vi "finalI.vi"() -> ()   [LabVIEW 2013]
panel:
  out "Array":i32[](array[numeric])
  out "appended array":i32[][](array[numeric])
  out "unsigned byte array":u8[](array[numeric])
  out "concatenated string":string
  out "we array":i32[](array[numeric])
  out "2d array sorted":i32[][](array[numeric])
  in  "stop":bool
  out "iterarions :":dbl
  out "Slide":u32(slide) scale=0.0..3000.0
  out "A letter":string
  out "B letter":string
  out "PASSWORD":string
  out "Utterance":dbl[](graph)
  out "Input Signal Energy":dbl
  out "?":bool
  out "?":bool
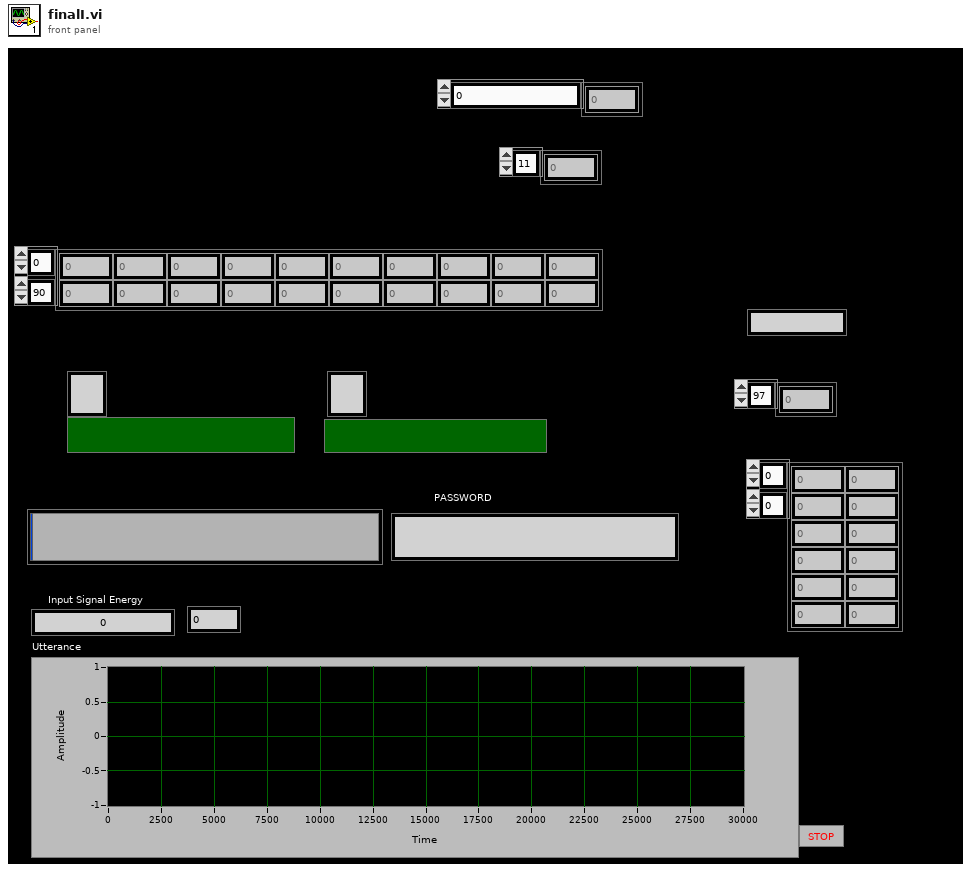
[diagram p1: front panel]
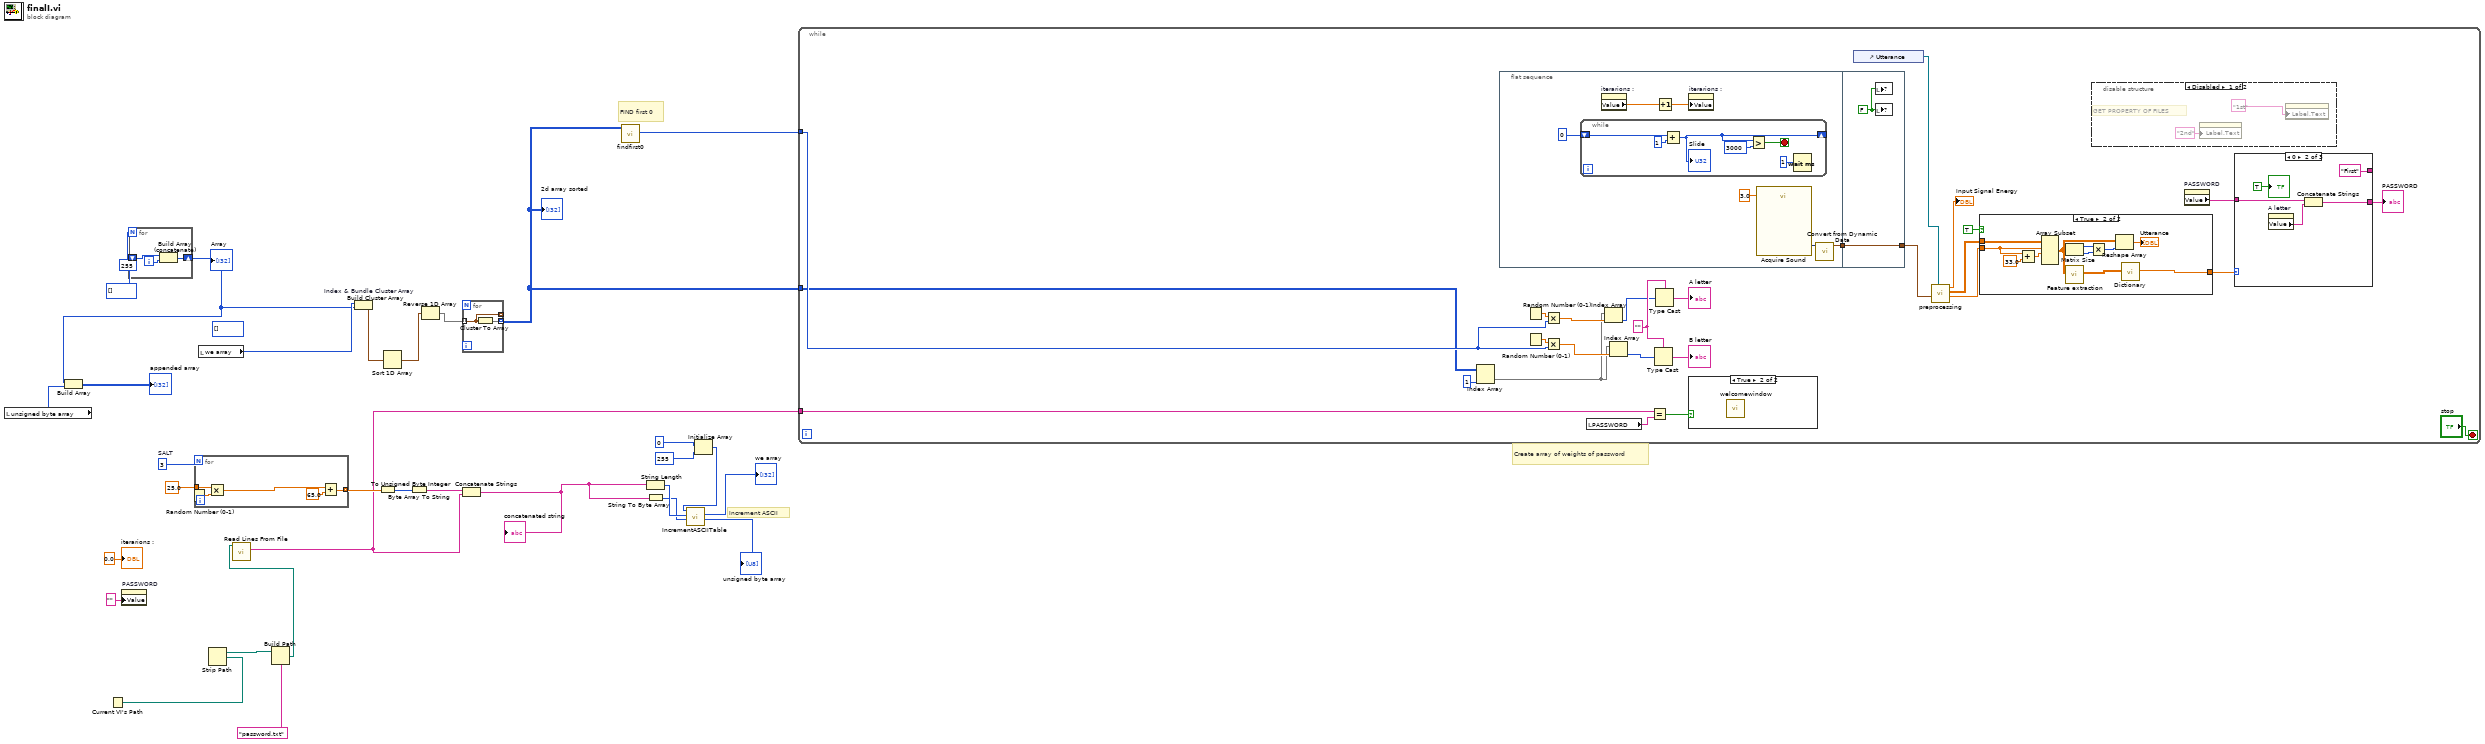
[diagram p0: block diagram]
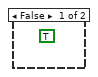
[diagram p3: hidden frame]
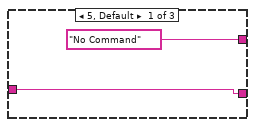
[diagram p4: hidden frame]
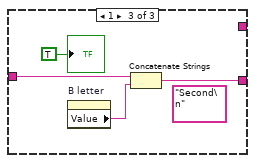
[diagram p5: hidden frame]
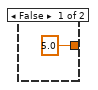
[diagram p6: hidden frame]
diagram:
  (unwired) i32[] []
  w26 = 3  # SALT
  # "FIND first 0"
  # "Create array of weights of password"
  # "Increment ASCII"
  n1 = local read "unsigned byte array"() -> (w9:u8[])
  n2 = Current VI's Path() -> (path=w4:path)
  n3 = property on="PASSWORD" class="Str"("Value"="" ("PASSWORD")) -> ()  [unwired: 2 in, 2 out]
  n4 = for {
    N: 255 -> [_]
    shift-right: [w31] -> w10
    shift-left: i32[] [] -> [w33]
    i -> [w32]
    n5 = Build Array (concatenate)(w33, w32) -> (w31:i32[])
  }
  "Array" <- w10
  n6 = Build Array(w10, w9) -> (→"appended array":i32[][])
  n7 = for {
    N: w26 -> [_]
    tunnel: 25.0 -> [w35]
    tunnel: [w34] -> w28 mode=indexing
    n8 = Random Number (0-1)() -> (number: 0 to 1=w38:dbl)
    n9 = Multiply(x=w35, y=w38) -> (x*y=w36:dbl)
    n10 = Add(x=w36, y=65.0) -> (x+y=w34:dbl)
  }
  n11 = local read "we array"() -> (w14:i32[])
  n12 = Strip Path(path=w4) -> (stripped path=w3:path)  [unwired: 1 out]
  n13 = Build Path(base path=w3, name or relative path="password.txt") -> (appended path=w1:path)
  n14 = call <vilib>:"Read Lines From File.vi"("file path (dialog if empty)"=w1) -> ("line string"=w5:string)  [unwired: 5 in, 3 out]
  n15 = Build Cluster Array "Index & Bundle Cluster Array"(w14, w10) -> (w15:cluster{"dimension size":i32, i32}[])
  n16 = To Unsigned Byte Integer(number=w28) -> (unsigned 8bit integer=w29:u8[])
  n17 = Sort 1D Array(array=w15) -> (sorted array=w13:cluster{"dimension size":i32, i32}[])
  n18 = Byte Array To String(unsigned byte array=w29) -> (string=w25:string)
  n19 = Reverse 1D Array(array=w13) -> (reversed array=w12:cluster{"dimension size":i32, i32}[])
  n20 = for {
    tunnel: [w39] -> _ mode=indexing
    tunnel: [w40] -> w7 mode=indexing
    tunnel: w12 -> [w39] mode=indexing
    n21 = Cluster To Array(cluster=w39) -> (array=w40:i32[])
  }
  "2d array sorted" <- w7
  n22 = Concatenate Strings(w25, w5) -> (w30:string)
  "concatenated string" <- w30
  n23 = call "findfirst0.vi"("Array"=w7) -> ("index of element"=w6:i32)  [unwired: 10 in]
  n24 = String Length(string=w30) -> (length=w24:i32)
  n25 = String To Byte Array(string=w30) -> (unsigned byte array=w21:u8[])
  "unsigned byte array" <- w21
  n26 = Initialize Array(0 ("dimension size"), 255 ("dimension size")) -> (w11:i32[])
  n27 = call "IncrementASCIITable.vi"("0255array"=w21, "Numeric"=w24, "Array in"=w11) -> ("we array"=→"we array":i32[])  [unwired: 7 in, 1 out]
  n28 = while {
    tunnel: w5 -> [w54]
    tunnel: w7 -> [w45]
    tunnel: w6 -> [w46]
    stop <- "stop" stop-if-true
    w49 = "" ("type")
    n29 = Index Array(array=w45, index (col)=1 ("disabled index (col)")) -> (element=w42:i32[])  [unwired: 1 in]
    n30 = flat-sequence {
      tunnel: [w97] -> w64
      tunnel: [w106] -> w62
      tunnel: w64 -> [w106]
      frame #0 {
        n31 = while {
          shift-right: [w101] -> _
          shift-left: u32 0 -> [w104]
          stop <- w99 stop-if-true
          n32 = Add(x=w104, y=1) -> (x+y=w101:u32)
          "Slide" <- w101
          n33 = Greater?(x=w101, y=u32 3000) -> (0:w99:bool)
          n34 = Wait (ms)(milliseconds to wait=u32 1) -> ()  [unwired: 1 out]
        }
        n35 = property on="iterarions :" class="DigNum (strict)"() -> ("Value"=w95:dbl)  [unwired: 2 in, 2 out]
        n36 = Increment(x=w95) -> (x+1=w94:dbl)
        n37 = property on="iterarions :" class="DigNum (strict)"("Value"=w94) -> ()  [unwired: 2 in, 2 out]
        n38 = call "Acquire Sound"("Duration (s)"=3.0) -> ("Data"=w98:dynamicdata)  [unwired: 17 in, 1 out]
        n39 = call "Convert from Dynamic Data"("Dynamic Data Type"=w98) -> ("Array of Waveform"=w97:waveform(dbl)[])  [unwired: 3 in]
      }
      frame #1 {
        w105 = FALSE
        n40 = local write item#?(w105) -> ()
        n41 = local write item#1(w105) -> ()
      }
    }
    n42 = Random Number (0-1)() -> (number: 0 to 1=w53:dbl)
    n43 = Random Number (0-1)() -> (number: 0 to 1=w52:dbl)
    n44 = Multiply(x=w53, y=w46) -> (x*y=w43:dbl)
    n45 = Multiply(x=w52, y=w46) -> (x*y=w51:dbl)
    n46 = local read "PASSWORD"() -> (w58:string)
    n47 = Index Array(array=w42, index=w43) -> (element=w41:i32)
    n48 = Index Array(array=w42, index=w51) -> (element=w48:i32)
    n49 = Equal?(x=w54, y=w58) -> (x = y?=w60:bool)
    n50 = Type Cast(type=w49, x=w48) -> (*(type *) &x=→"B letter":string)
    n51 = Type Cast(type=w49, x=w41) -> (*(type *) &x=→"A letter":string)
    n52 = case shown="True" w60 {
      frame False {
        (unwired) TRUE ("Boolean 2")
      }
      frame True {
        n53 = call "welcomewindow.vi"() -> ()  [unwired: 12 in]
      }
    }
    n54 = control-ref of="Utterance"() -> (w61:refnum<vi>)
    n55 = call "preprocessing.vi"("WaveformGraph in"=w61, "Input Speech"=w62) -> ("Start index"=w67:dbl, "Frames"=w66:dbl[][], "Signal energy"=→"Input Signal Energy":dbl)  [unwired: 6 in, 1 out]
    n56 = case shown="True" TRUE {
      tunnel: w67 -> [_ w85]
      tunnel: w66 -> [_ w86]
      tunnel: [5.0 ("Best Match") w84] -> w65
      frame False {
      }
      frame True {
        n57 = Add(x=w85, y=33.0 ("x")) -> (x+y=w91:dbl)
        n58 = Array Subset(array=w86, index (row)=w85, length (row)=w91) -> (w83:dbl[][])  [unwired: 2 in]
        n59 = Matrix Size(0:w83) -> (1:w90:i32, 2:w89:i32)
        n60 = call "Feature extraction.vi"("Utterance Frames"=w83) -> ("Acoustic vector"=w82:dbl[][])  [unwired: 10 in]
        n61 = Multiply(x=w90, y=w89) -> (x*y=w88:i32)
        n62 = Reshape Array(w83, w88) -> (→"Utterance":dbl[])
        n63 = call "Dictionary.vi"("Match Input"=w82) -> ("Best Match"=w84:dbl)  [unwired: 10 in]
      }
    }
    n64 = disable-structure shown="Disabled" {
      frame Disabled {
        # "GET PROPERTY OF FILES"
        n65 = property class="Bool (strict)"("Label.Text"="2nd") -> ()  [unwired: 2 in, 2 out]
        n66 = property class="Bool (strict)"("Label.Text"="1st" ("Caption.Text")) -> ()  [unwired: 2 in, 2 out]
      }
      frame Enabled {
      }
    }
    n67 = property on="PASSWORD" class="Str"() -> ("Value"=w59:string)  [unwired: 2 in, 2 out]
    n68 = case shown="0" w65 {
      tunnel: ["No Command" ("Command") "First" ("Command") _] -> _
      tunnel: [w70 w74 w79] -> w57
      tunnel: w59 -> [w70 w73 w78]
      frame 5, Default {
      }
      frame 0 {
        n69 = property on="A letter" class="Str"() -> ("Value"=w72:string)  [unwired: 2 in, 2 out]
        n70 = Concatenate Strings(w73, w72) -> (w74:string)
        "?" <- TRUE ("RIGHT")
      }
      frame 1 {
        (unwired) "Second\n" ("Command")
        n71 = property on="B letter" class="Str"() -> ("Value"=w77:string)  [unwired: 2 in, 2 out]
        n72 = Concatenate Strings(w78, w77) -> (w79:string)
        "?" <- TRUE ("RIGHT")
      }
    }
    "PASSWORD" <- w57
  }
  "iterarions :" <- 0.0 ("Numeric")
